vi "SavePlotData.vi"(8 "error in (no error)":errorcluster caption="错误输入（无错误）", 10 "数据输入":cluster{"数组":dbl[], "数组":dbl[]}, 11 "XYPlot 输入":refnum<class "XYPlot.lvclass">) -> (0 "error out":errorcluster caption="错误输出", 3 "XYPlot 输出":refnum<class "XYPlot.lvclass">)   [LabVIEW 2018, in "DataDisplay.lvlib" / "XYPlot.lvclass"]
uses:
  XYPlot.lvclass
  XYPlot.lvclass/XYPlot.ctl
  SubVI/WriteDataFile.vi
  DataDisplay.lvlib
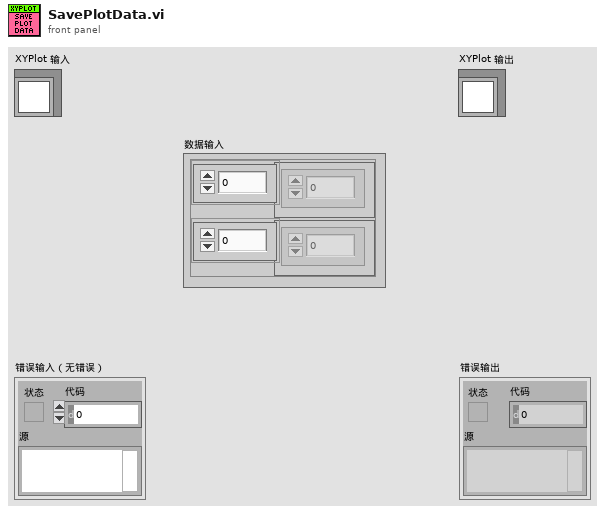
[diagram p1: front panel]
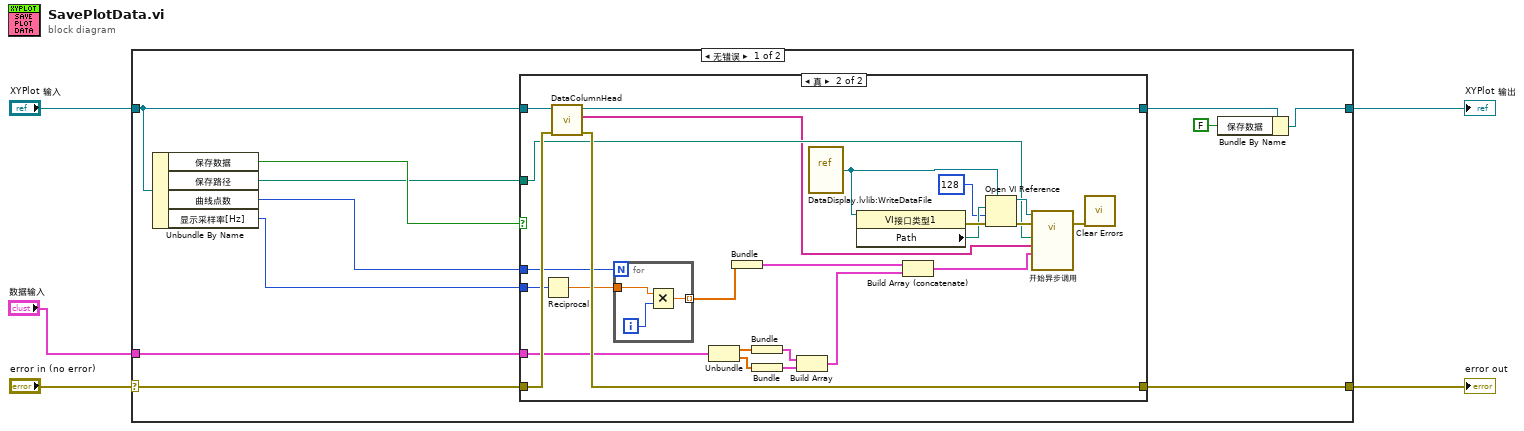
[diagram p0: block diagram]
diagram:
  n1 = case shown="无错误" "error in (no error)" {
    selector: "error in (no error)" -> [w10 w48]
    tunnel: [w9 w48] -> w4
    tunnel: [w11 w47] -> w2
    tunnel: "XYPlot 输入" -> [w13 w47]
    tunnel: "数据输入" -> [w8 _]
    frame No Error {
      n2 = Unbundle By Name(w13) -> ("保存数据"=w16:bool, "保存路径"=w14:path, "曲线点数"=w6:i32, "显示采样率[Hz]"=w7:i32)
      n3 = case shown="真" w16 {
        tunnel: w14 -> [_ w33]
        tunnel: [w17 w42] -> w12
        tunnel: w13 -> [w17 w43]
        tunnel: [w18 w40] -> w9
        tunnel: w10 -> [w18 w41]
        tunnel: w8 -> [_ w25]
        tunnel: w7 -> [_ w21]
        tunnel: w6 -> [_ w20]
        frame False {
        }
        frame True {
          n4 = Reciprocal(x=w21) -> (1/x=w22:dbl)
          n5 = call "DataColumnHead.vi"("error in (no error)"=w41, "XYPlot 输入"=w43) -> ("error out"=w40:errorcluster, "首行"=w32:string[], "XYPlot 输出"=w42:refnum<class "XYPlot.lvclass">)  [unwired: 7 in]
          n6 = for {
            N: w20 -> [_]
            tunnel: w22 -> [w45]
            tunnel: [w44] -> w23 mode=indexing
            i -> [w46]
            n7 = Multiply(x=w45, y=w46) -> (x*y=w44:dbl)
          }
          n8 = Unbundle(w25) -> ("数组"=w26:dbl[], "数组"=w27:dbl[])
          n9 = Bundle(w23) -> (w19:cluster{dbl[]})  [unwired: 1 in]
          n10 = Bundle("数组"=w26) -> (w28:cluster{"数组":dbl[]})  [unwired: 1 in]
          n11 = Bundle("数组"=w27) -> (w29:cluster{"数组":dbl[]})  [unwired: 1 in]
          n12 = Build Array(w28, w29) -> (w24:cluster{"数组":dbl[]}[])
          n13 = vi-ref "DataDisplay.lvlib:WriteDataFile.vi"() -> (w38:refnum<vi>)
          n14 = property class="VI接口类型1"(reference=w38) -> (error out=w39:errorcluster, "Path"=w37:path)  [unwired: 1 in, 1 out]
          n15 = Build Array (concatenate)(w19, w24) -> (w30:cluster{"数组":dbl[]}[])
          n16 = Open VI Reference(type specifier VI Refnum (for type only)=w38, vi path=w37, options=128 ("选项"), error in (no error)=w39) -> (vi reference=w35:refnum<vi>, error out=w34:errorcluster)  [unwired: 2 in]
          n17 = call-by-ref "开始异步调用"(reference=w35, error in=w34, "数据输入"=w30, "首行"=w32, "保存路径"=w33) -> (error out=w31:errorcluster)  [unwired: 9 in, 1 out]
          n18 = call <vilib>:"Clear Errors.vi"("error in (no error)"=w31) -> ()  [unwired: 5 in, 2 out]
        }
      }
      n19 = Bundle By Name(cluster=w12, "保存数据"=FALSE) -> (w11:refnum<class "XYPlot.lvclass">)
    }
    frame Error {
    }
  }
  "error out" <- w4
  "XYPlot 输出" <- w2
